vi "Acquisition next state logic.vi"(0 "Message Queues":T5, 5 "Acquired z-plane index":i32, 7 "Logging queue element":T1={"Imaging Protocol"=enum."Live Imaging", "Number of Trials"=0, "Frame Size"=512, "# Averaged frames"=0, "Dwell time (us)"=0.0, "Index of Z-plane"=0, "Timelapse?"=FALSE, "Logging process is active"=FALSE, "Speed logging enabled"=FALSE, "tdms file ref"=refnum, "path"=path "", "Trial Number"=0, "Expected # points acquired"=FALSE, "Manually stopped"=FALSE, "Last trial"=FALSE, "Ch0 data"=[], "Ch1 data"=[], "Ref Data"=[], "Ref Frame Time"=[], "Image Time"=[], "Continuous Time"=[], "Ref X Length"=0, "Ref Y Length"=0, "# Ref Averaged frames"=0, "Ref Dwell time (us)"=0.0, "Points acquired"={"Ch0 last trial"=0, "Ch1 last trial"=0, "All trials"=0}, "HW Timings File"=refnum} {"Ref Dwell time (us)" format="%#.6g"; "Frame Size" items=["100X100"=100, "128X128"=128, "200X200"=200, "256X256"=256, "512X512"=512, "1024x1024"=1024, "2048x2048"=2048]; "Dwell time (us)" format="%#.6g"}, 9 "Imaging Protocol":T2=enum."Live Imaging", 11 "error in":errorcluster) -> (6 "Index of next Z-plane to acquire":i32, 15 "error out":errorcluster)   [LabVIEW 2017]
uses:
  User Interface/Queue/Message Queue/Typedefs/All Message Queues.ctl
  User Interface/Queue/Message Queue/Typedefs/Message Cluster.ctl
  Typedefs/Logging queue element.ctl
  Typedefs/Imaging Protocols enum.ctl
  Typedefs/Frame Size.ctl
  Typedefs/Acquired points count.ctl
  Typedefs/Read Write Enum.ctl
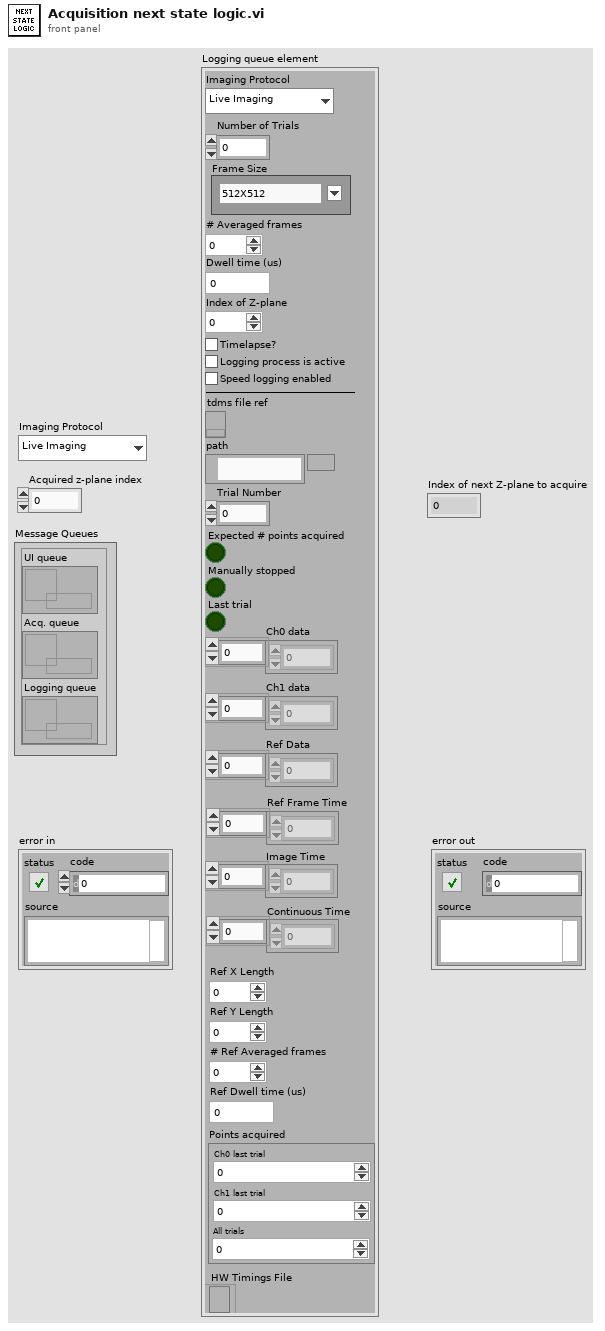
[diagram p1: front panel]
types:
  T1 = typedef "Logging queue element.ctl" = cluster{"Imaging Protocol":T2, "Number of Trials":u16, "Frame Size":T3, "# Averaged frames":u16, "Dwell time (us)":dbl, "Index of Z-plane":i32, "Timelapse?":bool, "Logging process is active":bool, "Speed logging enabled":bool, "tdms file ref":refnum<k34>, "path":path, "Trial Number":i32, "Expected # points acquired":bool, "Manually stopped":bool, "Last trial":bool, "Ch0 data":u32[], "Ch1 data":u32[], "Ref Data":u32[], "Ref Frame Time":u64[], "Image Time":u64[], "Continuous Time":u64[], "Ref X Length":u16, "Ref Y Length":u16, "# Ref Averaged frames":u16, "Ref Dwell time (us)":dbl, "Points acquired":T4, "HW Timings File":refnum<file>}
  T2 = typedef "Imaging Protocols enum.ctl" = enum16{"AOL Z-Stack", "Motor Z Stack", "Functional Acquisition", "Single Plane Acquisition", "Volume Acquisition", "Live Imaging", "Live Plane Imaging", "Live Volume Imaging"}
  T3 = typedef "Frame Size.ctl" = u16
  T4 = typedef "Acquired points count.ctl" = cluster{"Ch0 last trial":u64, "Ch1 last trial":u64, "All trials":u64}
  T5 = typedef "All Message Queues.ctl" = cluster{"UI queue":refnum<queue>, "Acq. queue":refnum<queue>, "Logging queue":refnum<queue>}
  T6 = typedef "Read Write Enum.ctl" = enum16{"Read", "Write"}
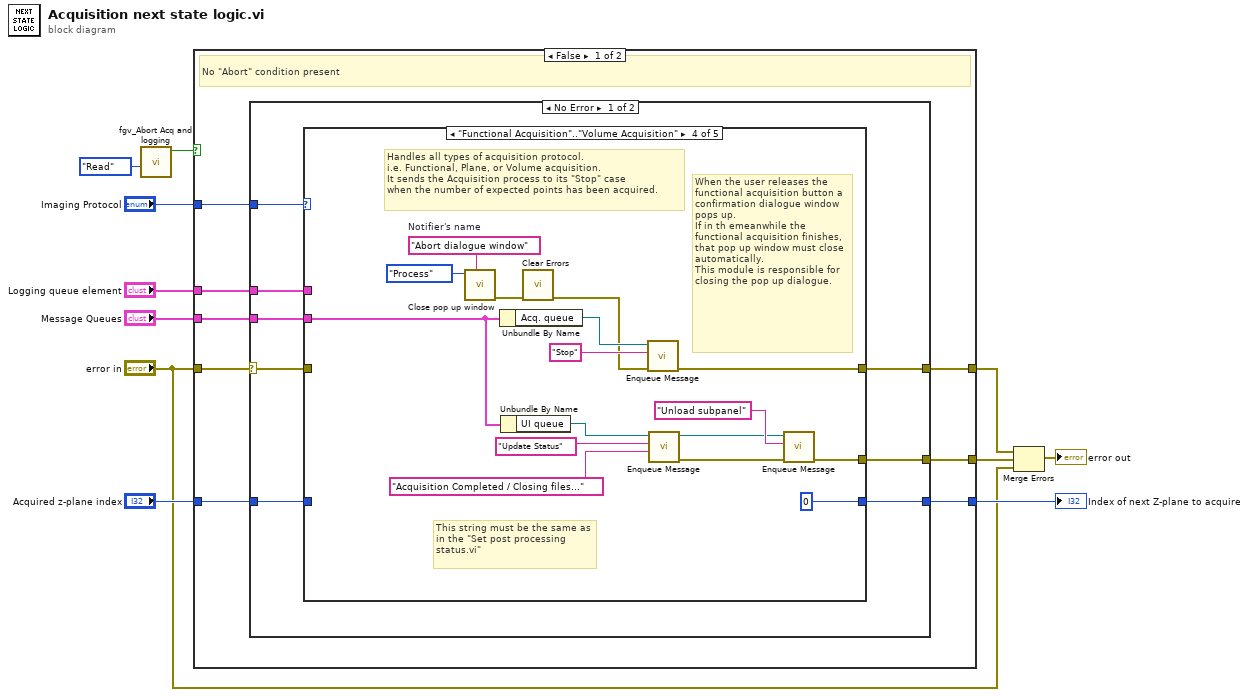
[diagram p0: block diagram]
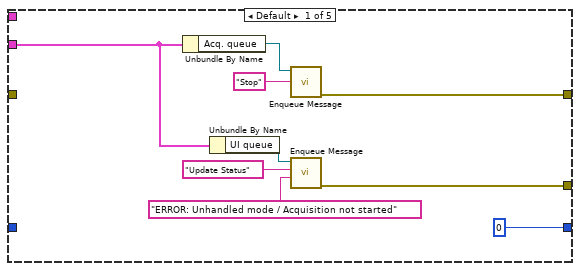
[diagram p2: hidden frame]
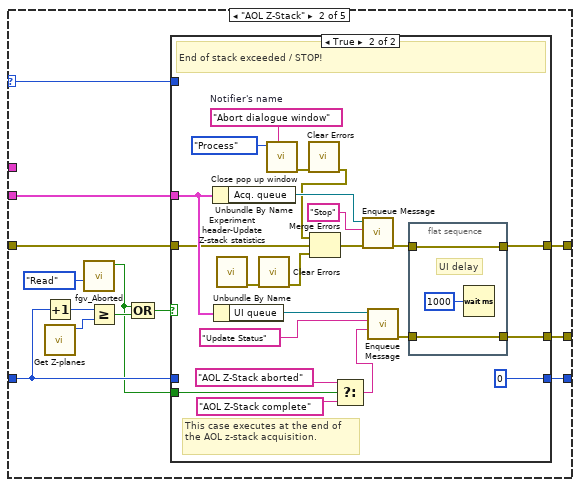
[diagram p3: hidden frame]
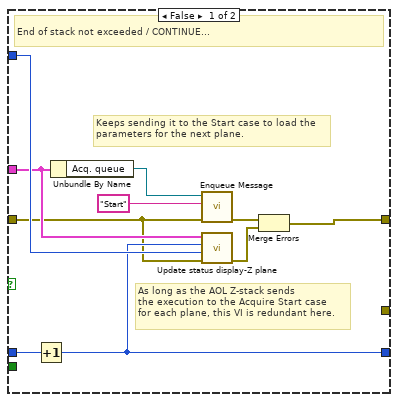
[diagram p4: hidden frame]
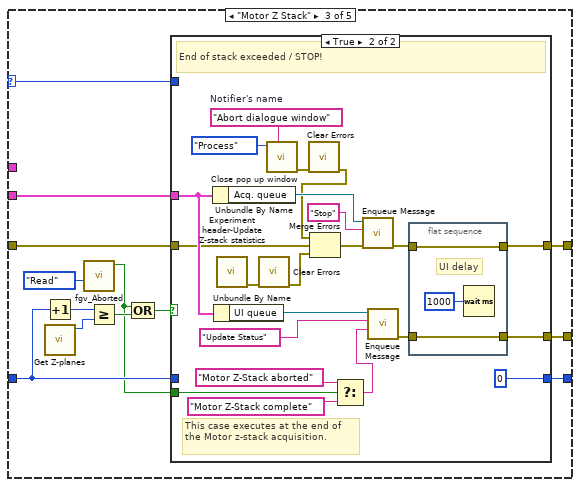
[diagram p5: hidden frame]
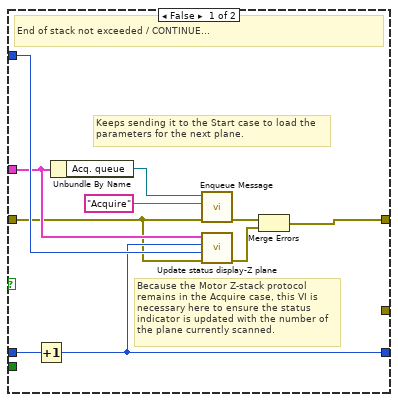
[diagram p6: hidden frame]
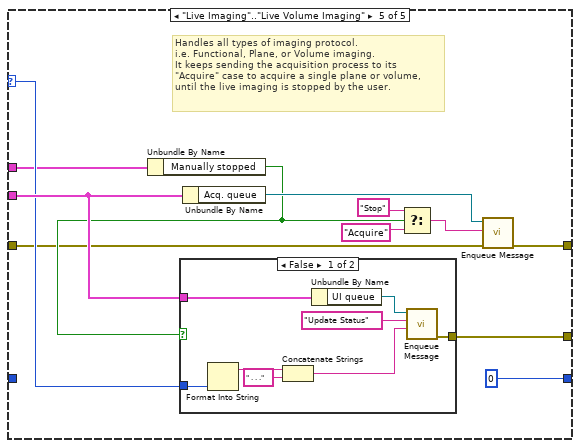
[diagram p7: hidden frame]
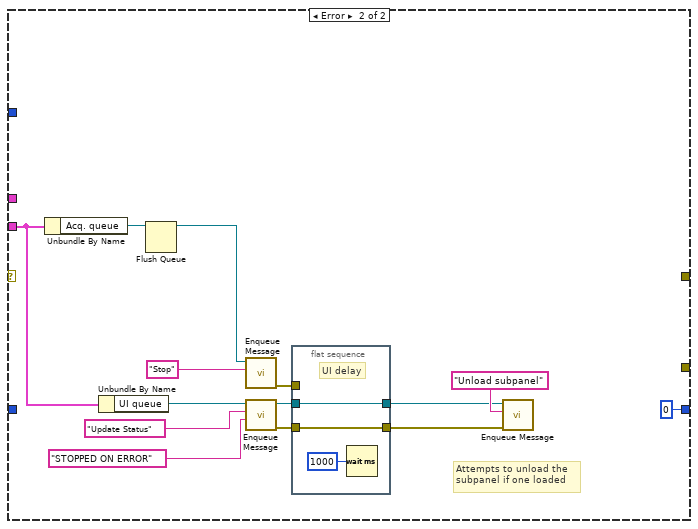
[diagram p9: hidden frame]
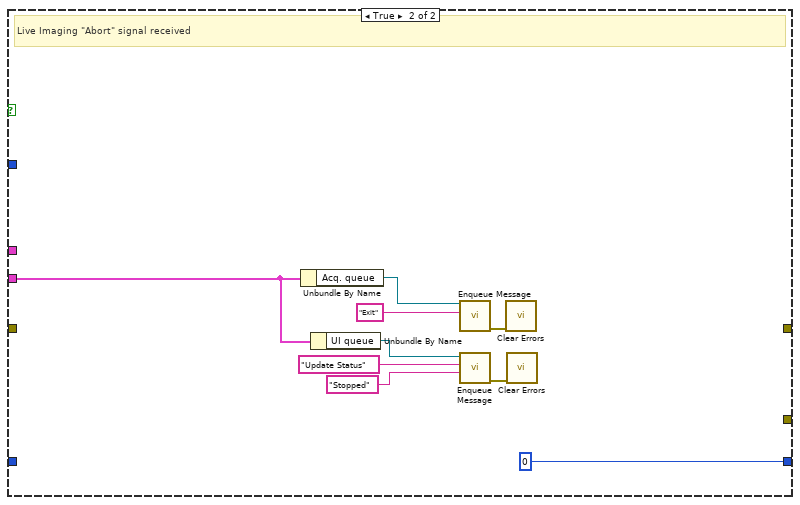
[diagram p10: hidden frame]
diagram:
  n1 = call "fgv_Abort Acq and logging.vi"("Function"=Read_Write_Enum."Read") -> ("Abort acquisition"=w1:bool)  [unwired: 9 in, 1 out]
  n2 = case shown="False" w1 {
    tunnel: [w19 _] -> w7
    tunnel: "error in" -> [w12 _]
    tunnel: [w18 0] -> w8
    tunnel: [w17 _] -> w6
    tunnel: "Acquired z-plane index" -> [w16 _]
    tunnel: "Imaging Protocol" -> [w14 _]
    tunnel: "Message Queues" -> [w15 w188]
    tunnel: "Logging queue element" -> [w13 _]
    frame False {
      # "No \"Abort\" condition present"
      n3 = case shown="No Error" w12 {
        selector: w12 -> [w20 _]
        tunnel: [w27 _] -> w19
        tunnel: [w26 0] -> w18
        tunnel: [w25 _] -> w17
        tunnel: w16 -> [w24 _]
        tunnel: w15 -> [w23 w173]
        tunnel: w14 -> [w22 _]
        tunnel: w13 -> [w21 _]
        frame No Error {
          n4 = case shown="\"Functional Acquisition\"..\"Volume Acquisition\"" w22 {
            selector: w22 -> [_ w41 w89 _ w157]
            tunnel: w20 -> [_ w44 w92 _ w150]
            tunnel: [w35 w48 w96 w147 w160] -> w27
            tunnel: [0 w46 w94 0 0] -> w26
            tunnel: w24 -> [_ w45 w93 _ _]
            tunnel: [w32 w47 w95 w139 w149] -> w25
            tunnel: w23 -> [w29 w43 w91 w143 w158]
            tunnel: w21 -> [_ _ _ _ w156]
            frame Default {
              n5 = Unbundle By Name(w29) -> ("Acq. queue"=w30:refnum<queue>)
              n6 = Unbundle By Name(w29) -> ("UI queue"=w31:refnum<queue>)
              n7 = call "Enqueue Message.vi"("Message"="Stop", "Queue"=w30) -> ("error out"=w35:errorcluster)  [unwired: 8 in, 1 out]
              n8 = call "Enqueue Message.vi"("Message Data"="ERROR: Unhandled mode / Acquisition not started" ("Message"), "Message"="Update Status", "Queue"=w31) -> ("error out"=w32:errorcluster)  [unwired: 7 in, 1 out]
            }
            frame "AOL Z-Stack" {
              n9 = Increment(x=w45) -> (x+1=w42:i32)
              n10 = call "Get Z-planes.vi"() -> ("# of Z-planes"=w49:i32)  [unwired: 7 in, 4 out]
              n11 = call "fgv_Aborted.vi"("Function"=Read_Write_Enum."Read") -> ("Funct Acq Aborted?"=w37:bool)  [unwired: 9 in, 1 out]
              n12 = Greater Or Equal?(x=w42, y=w49) -> (x >= y?=w39:bool)
              n13 = Compound Arithmetic op=OR(w37, w39) -> (w38:bool)
              n14 = case shown="True" w38 {
                tunnel: [w50 w74] -> w48
                tunnel: w44 -> [w53 w68]
                tunnel: w45 -> [w58 _]
                tunnel: [w54 0] -> w46
                tunnel: [_ w72] -> w47
                tunnel: w43 -> [w55 w78]
                tunnel: w41 -> [w56 _]
                tunnel: w37 -> [_ w60]
                frame False {
                  # "As long as the AOL Z-stack sends\nthe execution to the Acquire Start case\nfor each plane, this VI is redundant here."
                  # "Keeps sending it to the Start case to load the\nparameters for the next plane."
                  # "End of stack not exceeded / CONTINUE..."
                  n15 = Increment(x=w58) -> (x+1=w54:i32)
                  n16 = Unbundle By Name(w55) -> ("Acq. queue"=w57:refnum<queue>)
                  n17 = call "Enqueue Message.vi"("error in (no error)"=w53, "Message"="Start", "Queue"=w57) -> ("error out"=w51:errorcluster)  [unwired: 7 in, 1 out]
                  n18 = call "Update status display-Z plane.vi"("error in (no error)"=w53, "Imaging Protocol"=w56, "Acquired z-plane index"=w54, "Message Queues"=w55) -> ("error out"=w52:errorcluster)  [unwired: 7 in]
                  n19 = Merge Errors(w51, w52) -> (w50:errorcluster)
                }
                frame True {
                  w66 = "Abort dialogue window"  # Notifier's name
                  # "This case executes at the end of the AOL z-stack acquisition."
                  # "End of stack exceeded / STOP!"
                  n20 = Unbundle By Name(w78) -> ("Acq. queue"=w79:refnum<queue>)
                  n21 = Unbundle By Name(w78) -> ("UI queue"=w77:refnum<queue>)
                  n22 = call "Experiment header-Update Z-stack statistics.vi"() -> ("error out"=w71:errorcluster)  [unwired: 11 in]
                  n23 = call <vilib>:"Clear Errors.vi"("error in (no error)"=w71) -> ("error out"=w70:errorcluster)  [unwired: 5 in, 1 out]
                  n24 = call <userlib>:"Close pop up window.vi"("Notifier's name"=w66, "Location"=enum16{"Window", "Process"}."Process") -> ("error out"=w65:errorcluster)  [unwired: 7 in, 2 out]
                  n25 = call <vilib>:"Clear Errors.vi"("error in (no error)"=w65) -> ("error out"=w64:errorcluster)  [unwired: 5 in, 1 out]
                  n26 = Merge Errors(w64, w68, w70) -> (w69:errorcluster)
                  n27 = Select(t="AOL Z-Stack aborted" ("Message"), s=w60, f="AOL Z-Stack complete" ("Message")) -> (s? t:f=w62:string)
                  n28 = call "Enqueue Message.vi"("error in (no error)"=w69, "Message"="Stop", "Queue"=w79) -> ("error out"=w75:errorcluster)  [unwired: 7 in, 1 out]
                  n29 = call "Enqueue Message.vi"("Message Data"=w62, "Message"="Update Status", "Queue"=w77) -> ("error out"=w73:errorcluster)  [unwired: 7 in, 1 out]
                  n30 = flat-sequence {
                    tunnel: w75 -> [w83]
                    tunnel: [w83] -> w74
                    tunnel: w73 -> [w82]
                    tunnel: [w82] -> w72
                    frame #0 {
                      # "UI delay"
                      n31 = Wait (ms)(milliseconds to wait=u32 1000) -> ()  [unwired: 1 out]
                    }
                  }
                }
              }
            }
            frame "Motor Z Stack" {
              n32 = Increment(x=w93) -> (x+1=w90:i32)
              n33 = call "Get Z-planes.vi"() -> ("# of Z-planes"=w97:i32)  [unwired: 7 in, 4 out]
              n34 = call "fgv_Aborted.vi"("Function"=Read_Write_Enum."Read") -> ("Funct Acq Aborted?"=w85:bool)  [unwired: 9 in, 1 out]
              n35 = Greater Or Equal?(x=w90, y=w97) -> (x >= y?=w87:bool)
              n36 = Compound Arithmetic op=OR(w85, w87) -> (w86:bool)
              n37 = case shown="True" w86 {
                tunnel: [w98 w122] -> w96
                tunnel: w92 -> [w101 w116]
                tunnel: w93 -> [w106 _]
                tunnel: [w102 0] -> w94
                tunnel: [_ w120] -> w95
                tunnel: w91 -> [w103 w126]
                tunnel: w89 -> [w104 _]
                tunnel: w85 -> [_ w108]
                frame False {
                  # "Because the Motor Z-stack protocol\nremains in the Acquire case, this VI is necessary here to ensure the status indicator is updated with the number of the plane currently scanned."
                  # "Keeps sending it to the Start case to load the\nparameters for the next plane."
                  # "End of stack not exceeded / CONTINUE..."
                  n38 = Increment(x=w106) -> (x+1=w102:i32)
                  n39 = Unbundle By Name(w103) -> ("Acq. queue"=w105:refnum<queue>)
                  n40 = call "Enqueue Message.vi"("error in (no error)"=w101, "Message"="Acquire", "Queue"=w105) -> ("error out"=w99:errorcluster)  [unwired: 7 in, 1 out]
                  n41 = call "Update status display-Z plane.vi"("error in (no error)"=w101, "Imaging Protocol"=w104, "Acquired z-plane index"=w102, "Message Queues"=w103) -> ("error out"=w100:errorcluster)  [unwired: 7 in]
                  n42 = Merge Errors(w99, w100) -> (w98:errorcluster)
                }
                frame True {
                  w114 = "Abort dialogue window"  # Notifier's name
                  # "This case executes at the end of the Motor z-stack acquisition."
                  # "End of stack exceeded / STOP!"
                  n43 = Unbundle By Name(w126) -> ("Acq. queue"=w127:refnum<queue>)
                  n44 = Unbundle By Name(w126) -> ("UI queue"=w125:refnum<queue>)
                  n45 = call "Experiment header-Update Z-stack statistics.vi"() -> ("error out"=w119:errorcluster)  [unwired: 11 in]
                  n46 = call <vilib>:"Clear Errors.vi"("error in (no error)"=w119) -> ("error out"=w118:errorcluster)  [unwired: 5 in, 1 out]
                  n47 = call <userlib>:"Close pop up window.vi"("Notifier's name"=w114, "Location"=enum16{"Window", "Process"}."Process") -> ("error out"=w113:errorcluster)  [unwired: 7 in, 2 out]
                  n48 = call <vilib>:"Clear Errors.vi"("error in (no error)"=w113) -> ("error out"=w112:errorcluster)  [unwired: 5 in, 1 out]
                  n49 = Merge Errors(w112, w116, w118) -> (w117:errorcluster)
                  n50 = Select(t="Motor Z-Stack aborted" ("Message"), s=w108, f="Motor Z-Stack complete" ("Message")) -> (s? t:f=w110:string)
                  n51 = call "Enqueue Message.vi"("error in (no error)"=w117, "Message"="Stop", "Queue"=w127) -> ("error out"=w123:errorcluster)  [unwired: 7 in, 1 out]
                  n52 = call "Enqueue Message.vi"("Message Data"=w110, "Message"="Update Status", "Queue"=w125) -> ("error out"=w121:errorcluster)  [unwired: 7 in, 1 out]
                  n53 = flat-sequence {
                    tunnel: w123 -> [w131]
                    tunnel: [w131] -> w122
                    tunnel: w121 -> [w130]
                    tunnel: [w130] -> w120
                    frame #0 {
                      # "UI delay"
                      n54 = Wait (ms)(milliseconds to wait=u32 1000) -> ()  [unwired: 1 out]
                    }
                  }
                }
              }
            }
            frame "Functional Acquisition".."Volume Acquisition" {
              w136 = "Abort dialogue window"  # Notifier's name
              # "When the user releases the functional acquisition button a confirmation dialogue window pops up.\nIf in th emeanwhile the functional acquisition finishes, that pop up window must close automatically.\nThis module is responsible for closing the pop up dialogue."
              # "This string must be the same as in the \"Set post processing status.vi\""
              # "Handles all types of acquisition protocol.\ni.e. Functional, Plane, or Volume acquisition.\nIt sends the Acquisition process to its \"Stop\" case\nwhen the number of expected points has been acquired."
              n55 = call <userlib>:"Close pop up window.vi"("Notifier's name"=w136, "Location"=enum16{"Window", "Process"}."Process") -> ("error out"=w134:errorcluster)  [unwired: 7 in, 2 out]
              n56 = Unbundle By Name(w143) -> ("Acq. queue"=w144:refnum<queue>)
              n57 = Unbundle By Name(w143) -> ("UI queue"=w142:refnum<queue>)
              n58 = call <vilib>:"Clear Errors.vi"("error in (no error)"=w134) -> ("error out"=w133:errorcluster)  [unwired: 5 in, 1 out]
              n59 = call "Enqueue Message.vi"("error in (no error)"=w133, "Message"="Stop", "Queue"=w144) -> ("error out"=w147:errorcluster)  [unwired: 7 in, 1 out]
              n60 = call "Enqueue Message.vi"("Message Data"="Acquisition Completed / Closing files..." ("Message"), "Message"="Update Status", "Queue"=w142) -> ("error out"=w140:errorcluster, "Queue out"=w138:refnum<queue>)  [unwired: 7 in]
              n61 = call "Enqueue Message.vi"("error in (no error)"=w140, "Message"="Unload subpanel", "Queue"=w138) -> ("error out"=w139:errorcluster)  [unwired: 7 in, 1 out]
            }
            frame "Live Imaging".."Live Volume Imaging" {
              # "Handles all types of imaging protocol.\ni.e. Functional, Plane, or Volume imaging.\nIt keeps sending the acquisition process to its\n\"Acquire\" case to acquire a single plane or volume,\nuntil the live imaging is stopped by the user."
              n62 = Unbundle By Name(w156) -> ("Manually stopped"=w151:bool)
              n63 = case shown="False" w151 {
                tunnel: w158 -> [w166 _]
                tunnel: w157 -> [w165 _]
                tunnel: [w162 _] -> w149
                frame False {
                  n64 = Format Into String(w165) -> (resulting string=w164:string)  [unwired: 3 in, 1 out]
                  n65 = Concatenate Strings(w164, " . . ." ("string")) -> (w161:string)
                  n66 = Unbundle By Name(w166) -> ("UI queue"=w167:refnum<queue>)
                  n67 = call "Enqueue Message.vi"("Message Data"=w161, "Message"="Update Status", "Queue"=w167) -> ("error out"=w162:errorcluster)  [unwired: 7 in, 1 out]
                }
                frame True {
                }
              }
              n68 = Unbundle By Name(w158) -> ("Acq. queue"=w159:refnum<queue>)
              n69 = Select(t="Stop" ("Message"), s=w151, f="Acquire" ("Message")) -> (s? t:f=w153:string)
              n70 = call "Enqueue Message.vi"("error in (no error)"=w150, "Message"=w153, "Queue"=w159) -> ("error out"=w160:errorcluster)  [unwired: 7 in, 1 out]
            }
          }
        }
        frame Error {
          # "Attempts to unload the\nsubpanel if one loaded"
          n71 = Unbundle By Name(w173) -> ("Acq. queue"=w182:refnum<queue>)
          n72 = Unbundle By Name(w173) -> ("UI queue"=w176:refnum<queue>)
          n73 = Flush Queue(queue=w182) -> (queue out=w174:refnum<queue>)  [unwired: 1 in, 2 out]
          n74 = call "Enqueue Message.vi"("Message"="Stop", "Queue"=w174) -> ("error out"=w179:errorcluster)  [unwired: 8 in, 1 out]
          n75 = call "Enqueue Message.vi"("Message Data"="STOPPED ON ERROR" ("Message"), "Message"="Update Status", "Queue"=w176) -> ("error out"=w180:errorcluster, "Queue out"=w170:refnum<queue>)  [unwired: 7 in]
          n76 = flat-sequence {
            tunnel: w179 -> [_]
            tunnel: w180 -> [w184]
            tunnel: [w184] -> w171
            tunnel: [w183] -> w169
            tunnel: w170 -> [w183]
            frame #0 {
              # "UI delay"
              n77 = Wait (ms)(milliseconds to wait=u32 1000) -> ()  [unwired: 1 out]
            }
          }
          n78 = call "Enqueue Message.vi"("error in (no error)"=w171, "Message"="Unload subpanel", "Queue"=w169) -> ()  [unwired: 7 in, 2 out]
        }
      }
    }
    frame True {
      # "Live Imaging \"Abort\" signal received"
      n79 = Unbundle By Name(w188) -> ("Acq. queue"=w192:refnum<queue>)
      n80 = Unbundle By Name(w188) -> ("UI queue"=w189:refnum<queue>)
      n81 = call "Enqueue Message.vi"("Message"="Exit", "Queue"=w192) -> ("error out"=w186:errorcluster)  [unwired: 8 in, 1 out]
      n82 = call "Enqueue Message.vi"("Message Data"="Stopped" ("Message"), "Message"="Update Status", "Queue"=w189) -> ("error out"=w187:errorcluster)  [unwired: 7 in, 1 out]
      n83 = call <vilib>:"Clear Errors.vi"("error in (no error)"=w186) -> ()  [unwired: 5 in, 2 out]
      n84 = call <vilib>:"Clear Errors.vi"("error in (no error)"=w187) -> ()  [unwired: 5 in, 2 out]
    }
  }
  "Index of next Z-plane to acquire" <- w8
  n85 = Merge Errors(w7, w6, "error in") -> (→"error out":errorcluster)
